vi "Asylum_Driver_TerminateLithographyObject.vi"(6 "Z Move Setpoint":dbl, 8 "error in (no error)":errorcluster, 11 "Application":refnum<k7>) -> (0 "error out":errorcluster, 3 "Application Out":refnum<k7>)   [LabVIEW 2019]
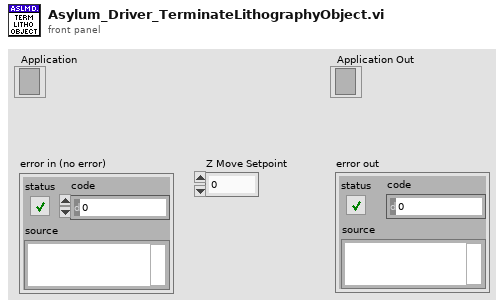
[diagram p1: front panel]
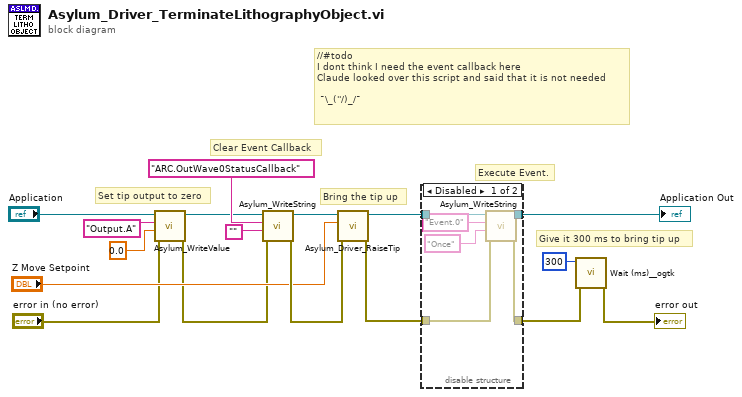
[diagram p0: block diagram]
diagram:
  # "//#todo\nI dont think I need the event callback here\nClaude looked over this script and said that it is not needed\n\n ¯\\_(''/)_/¯"
  # "Give it 300 ms to bring tip up"
  # "Execute Event."
  # "Bring the tip up"
  # "Clear Event Callback"
  # "Set tip output to zero"
  n1 = call <userlib>:"Asylum_WriteValue.vi"("error in (no error)"="error in (no error)", "value"=0.0, "parameterName"="Output.A", "Application"="Application") -> ("error out"=w3:errorcluster, "Application"=w4:refnum<k7>)  [unwired: 6 in]
  n2 = call <userlib>:"Asylum_WriteString.vi"("error in (no error)"=w3, "valueString"="", "parameterName"="ARC.OutWave0StatusCallback", "Application"=w4) -> ("error out"=w14:errorcluster, "Application"=w15:refnum<k7>)  [unwired: 6 in]
  n3 = call "Asylum_Driver_RaiseTip.vi"("error in (no error)"=w14, "Z Move Setpoint"="Z Move Setpoint", "Application In"=w15) -> ("error out"=w9:errorcluster, "Application Out"=w10:refnum<k7>)  [unwired: 7 in]
  n4 = disable-structure shown="Disabled" {
    disable-tunnel: [w23 w25] -> w12
    disable-tunnel: w10 -> [w22 w24]
    disable-tunnel: w9 -> [w18 w25]
    disable-tunnel: [w21 w24] -> w8
    frame Disabled {
      n5 = call <userlib>:"Asylum_WriteString.vi"("error in (no error)"=w18, "valueString"="Once", "parameterName"="Event.0", "Application"=w22) -> ("error out"=w23:errorcluster, "Application"=w21:refnum<k7>)  [unwired: 6 in]
    }
    frame Enabled {
    }
  }
  "Application Out" <- w8
  n6 = call <userlib>:"Wait (ms)__ogtk.vi"("error in (no error)"=w12, "milliseconds to wait"=u32 300) -> ("error out"=→"error out":errorcluster)  [unwired: 8 in, 1 out]
